vi "Sample.vi"() -> ()   [LabVIEW 2013]
panel:
  out "OK Done":bool=TRUE
  # "Sample program to show how to control SHOT-702 Stage controller."
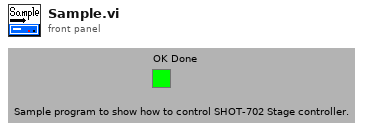
[diagram p1: front panel]
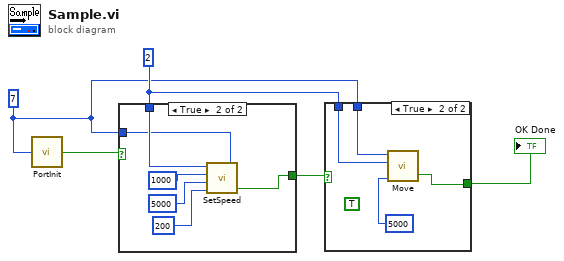
[diagram p0: block diagram]
diagram:
  w2 = 7
  w3 = 2
  n1 = call "PortInit.vi"("PortNumber"=w2) -> ("Done"=w1:bool)
  n2 = case shown="True" w1 {
    selector: w1 -> [w6 _]
    tunnel: [w6 w7] -> w4
    tunnel: w3 -> [_ w9]
    tunnel: w2 -> [_ w8]
    frame False {
    }
    frame True {
      n3 = call "SetSpeed.vi"("Port Number"=w8, "Acceleration Time"=200, "High Speed"=5000, "Low Speed"=1000, "Axis Number"=w9) -> ("OK Done"=w7:bool)  [unwired: 1 out]
    }
  }
  n4 = case shown="True" w4 {
    selector: w4 -> [w13 _]
    tunnel: [w13 w14] -> w5
    tunnel: w3 -> [_ w16]
    tunnel: w2 -> [_ w15]
    frame False {
    }
    frame True {
      (unwired) TRUE
      n5 = call "Move.vi"("Pulse Number"=5000, "Axis Number"=w16, "Port Number"=w15) -> ("OK Done"=w14:bool)  [unwired: 1 in, 1 out]
    }
  }
  "OK Done" <- w5
